vi "Opcode at last 2 positions.vi"(11 "Opcode":u16 format="%04x") -> (3 "00FF":u8 format="%02x")   [LabVIEW 2021]
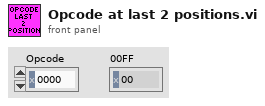
[diagram p1: front panel]
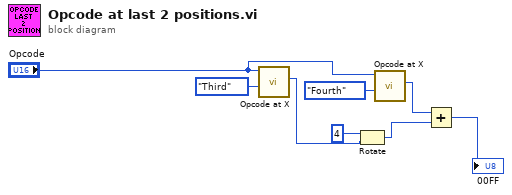
[diagram p0: block diagram]
diagram:
  n1 = call "Opcode at X.vi"("X Position"=enum16{"First", "Second", "Third", "Fourth"}."Third", "Opcode"="Opcode") -> ("Opcode at X Position (U8)"=w5:u8)  [unwired: 9 in]
  n2 = Rotate(1:w5, 2:i16 4 ("y")) -> (0:w6:u8)
  n3 = call "Opcode at X.vi"("X Position"=enum16{"First", "Second", "Third", "Fourth"}."Fourth", "Opcode"="Opcode") -> ("Opcode at X Position (U8)"=w3:u8)  [unwired: 9 in]
  n4 = Add(x=w3, y=w6) -> (x+y=→"00FF":u8)
